vi "Register Worker.vi"(8 "error in (no error)":errorcluster, 10 "Worker":refnum<class "Job Handler.lvclass">, 11 "Work Dispatcher In":refnum<class "Work Dispatcher.lvclass">) -> (0 "error out":errorcluster, 3 "Work Dispatcher Out":refnum<class "Work Dispatcher.lvclass">)   [LabVIEW 2021, in "Work Dispatcher.lvclass"]
uses:
  Work Dispatcher.lvclass
  <vilib>/Astemes/Triarc Framework/Process/Process.lvclass/Process.ctl
  <vilib>/Astemes/Triarc Framework/Process/Public/Lifecycle/Get Lifecycle State.vi
  <vilib>/Astemes/Triarc Framework/Process/Private/SubVIs/Handle Debug Data.vi
  <vilib>/Utility/error.llb/Clear Errors.vi
  <vilib>/Utility/High Resolution Relative Seconds.vi
  <vilib>/Utility/error.llb/Error Cluster From Error Code.vi
  Work Dispatcher.lvclass/Work Dispatcher.ctl
  <vilib>/Astemes/Triarc Framework/Process/Process.lvclass
  People/Process Job/Job Handler.lvclass
  C:/Program Files (x86)/National Instruments/LabVIEW 2021/vi.lib/Astemes/Triarc Framework/Process/Process.lvclass
  C:/Program Files (x86)/National Instruments/LabVIEW 2021/vi.lib/Astemes/Triarc Framework/Base/Base.lvclass
  C:/Program Files (x86)/National Instruments/LabVIEW 2021/vi.lib/Astemes/Triarc Framework/Error Handler Interface/Error Handler Interface.lvclass
  C:/Program Files (x86)/National Instruments/LabVIEW 2021/vi.lib/Astemes/Triarc Framework/Logging/Logging.lvclass
  C:/Git/astemes-triarc-examples/Coffee Shop/Processes/Work Dispatcher/Work Dispatcher.lvclass
  C:/Git/astemes-triarc-examples/Coffee Shop/Processes/People/Process Job/Job Handler.lvclass
  C:/Program Files (x86)/National Instruments/LabVIEW 2021/vi.lib/Astemes/Triarc Framework/Helper Loop/Helper Loop.lvclass
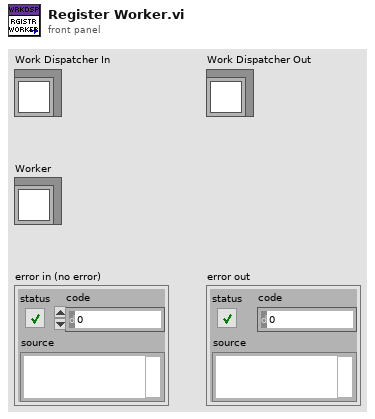
[diagram p1: front panel]
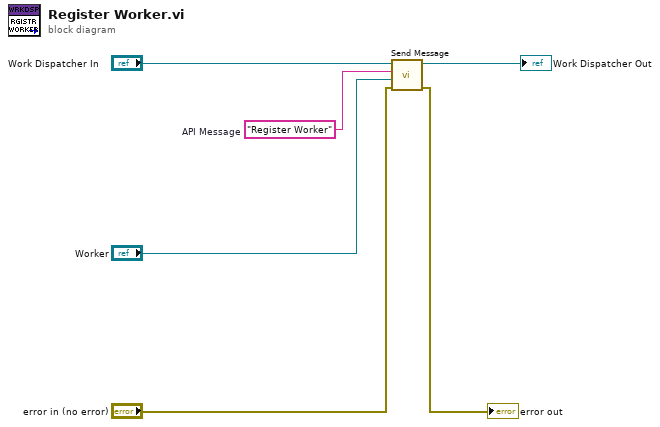
[diagram p0: block diagram]
diagram:
  w3 = "Register Worker"  # API Message
  n1 = call <vilib>:"Send Message.vi"("error in (no error)"="error in (no error)", "Message Data"="Worker", "Message"=w3, "Process In"="Work Dispatcher In") -> ("error out"=→"error out":errorcluster, "Process Out"=→"Work Dispatcher Out":refnum<class "Work Dispatcher.lvclass">)  [unwired: 6 in]
